vi "Get Clock History Map.vi"(8 "error in (no error)":errorcluster, 11 "CIFPluginManager in":refnum<class "CIFPluginManager.lvclass">) -> (0 "error out":errorcluster, 3 "Clock History Map":T1)   [LabVIEW 2021, in "CIFPluginManager.lvclass"]
uses:
  CIFPluginManager.lvclass
  CIFPluginManager.lvclass/CIFPluginManager.ctl
  <vilib>/CIF Foundation/CIF Utilities/Time/Typedef/Timestamp Pair.ctl
  <vilib>/CIF Foundation/CIF Utilities/Time/Time_CIF_U.lvlib
  <vilib>/CIF Foundation/CIF Utilities/Time/Typedef/Clock History.ctl
  <vilib>/CIF Foundation/CIF Utilities/Time/Typedef/Clock History Map.ctl
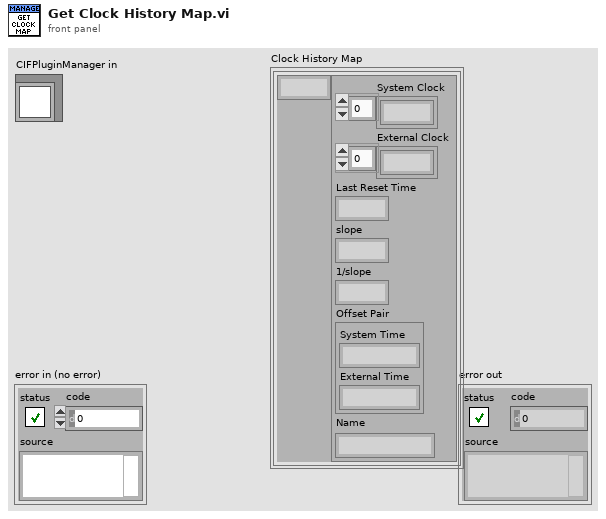
[diagram p1: front panel]
types:
  T1 = typedef "Time_CIF_U.lvlib/Clock History Map.ctl" = map{u8, T2}
  T2 = typedef "Time_CIF_U.lvlib/Clock History.ctl" = cluster{"System Clock":i64[], "External Clock":i64[], "Last Reset Time":i64, "slope":dbl, "1/slope":dbl, "Offset Pair":T3, "Name":string}
  T3 = typedef "Time_CIF_U.lvlib/Timestamp Pair.ctl" = cluster{"System Time":i64, "External Time":i64}
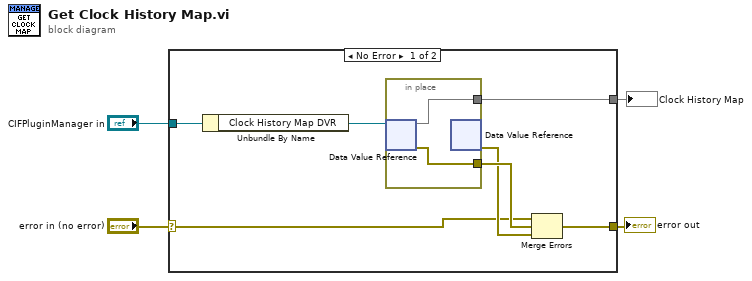
[diagram p0: block diagram]
diagram:
  n1 = case shown="No Error" "error in (no error)" {
    selector: "error in (no error)" -> [w7 w14]
    tunnel: [w6 w14] -> w3
    tunnel: "CIFPluginManager in" -> [w10 _]
    tunnel: [w5 _] -> w1
    frame No Error {
      n2 = Unbundle By Name(w10) -> ("Clock History Map DVR"=w11:refnum<data-value>)
      n3 = in-place {
        in-place-border: [w13] -> w5
        in-place-border: [w12] -> w9
        n4 = in-place-dvr #1(w11) -> (w13:T1, w12:errorcluster)
        n5 = in-place-dvr #1() -> (w8:errorcluster)  [unwired: 1 in, 1 out]
      }
      n6 = Merge Errors(w7, w9, w8) -> (w6:errorcluster)
    }
    frame Error {
    }
  }
  "error out" <- w3
  "Clock History Map" <- w1
